vi "Read From Spreadsheet File (DBL)-Modified.vi"(0 "file path (dialog if empty)":path, 1 "format (%.3f)":string="%.3f", 5 "number of rows (all:-1)":i32=-1, 9 "start of read offset (chars.:0)":i32, 11 "max characters/row  (no limit:0)":i32, 12 "transpose (no:F)":bool, 14 "delimiter (\\t)":string="\t") -> (3 "new file path (Not A Path if cancelled)":path, 4 "all rows":dbl[][](array[numeric]), 6 "first row":dbl[](array[numeric]), 8 "EOF?":bool, 10 "mark after read (chars.)":i32, 15 "error out":errorcluster)   [LabVIEW 2020]
doc: "Reads a specified number of lines or rows from a numeric text file beginning at a specified character offset and converts the data to a 2D, double-precision array of numbers, strings, or integers. You must manually select the polymorphic instance you want to use."
panel:
  in  "type (empty)":dbl[][](array[numeric])
  # "row\ncolumn"
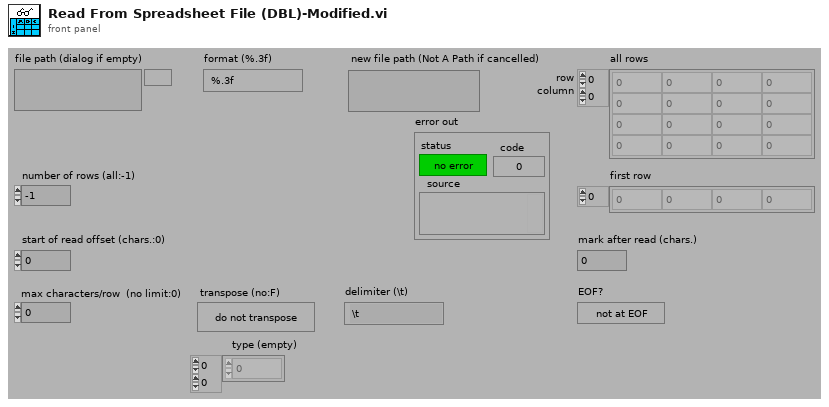
[diagram p1: front panel]
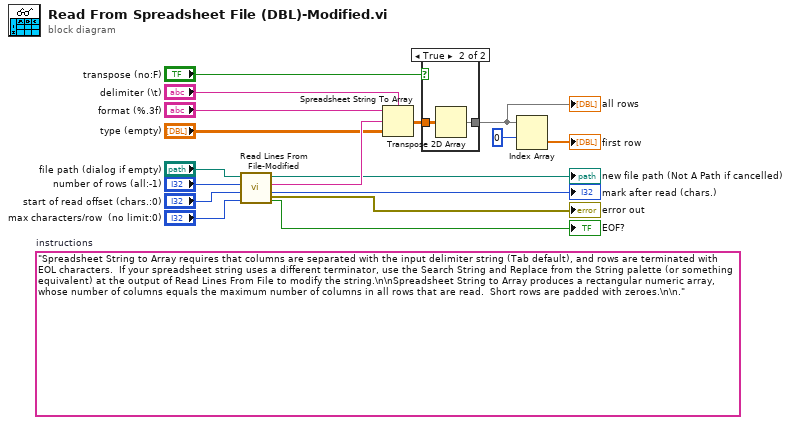
[diagram p0: block diagram]
diagram:
  (unwired) "Spreadsheet String to Array requires that columns are separated with the input delimiter string (Tab default), and rows are terminated with EOL characters.  If your spreadsheet string uses a different terminator, use the Search String and Replace from the String palette (or something equivalent) at the output of Read Lines From File to modify the string.\n\nSpreadsheet String to Array produces a rectangular numeric array, whose number of columns equals the maximum number of columns in all rows that are read.  Short rows are padded with zeroes.\n\n."  # instructions
  n1 = call "Read Lines From File-Modified.vi"("[max characters per line]  (no limit:0)"="max characters/row  (no limit:0)", "start of read offset (chars.:0)"="start of read offset (chars.:0)", "number of lines (all:-1)"="number of rows (all:-1)", "file path (dialog if empty)"="file path (dialog if empty)") -> ("EOF?"=→"EOF?":bool, "mark after read (chars.)"=→"mark after read (chars.)":i32, "line string"=w13:string, "new file path (Not A Path if cancelled)"=→"new file path (Not A Path if cancelled)":path, "error out"=→"error out":errorcluster)  [unwired: 3 in]
  n2 = Spreadsheet String To Array(delimiter (Tab)="delimiter (\\t)", format string="format (%.3f)", spreadsheet string=w13, array type (2D Dbl)="type (empty)") -> (array=w11:dbl[][])
  n3 = case shown="True" "transpose (no:F)" {
    tunnel: [w18 w20] -> w8
    tunnel: w11 -> [w18 w19]
    frame False {
    }
    frame True {
      n4 = Transpose 2D Array(2D array=w19) -> (transposed array=w20:dbl[][])
    }
  }
  "all rows" <- w8
  n5 = Index Array(array=w8, index (row)=0) -> (element=→"first row":dbl[])  [unwired: 1 in]
